vi "Calulate Rotation and Inclination.vi"(0 "Ch 0":dbl, 7 "Ch 1":dbl, 9 "Ch 2":dbl) -> (4 "Magnitude XYZ(g)":dbl, 8 "Inclination":dbl, 10 "Rotation":dbl)   [LabVIEW 2011]
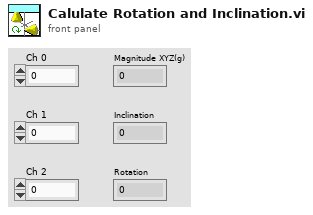
[diagram p1: front panel]
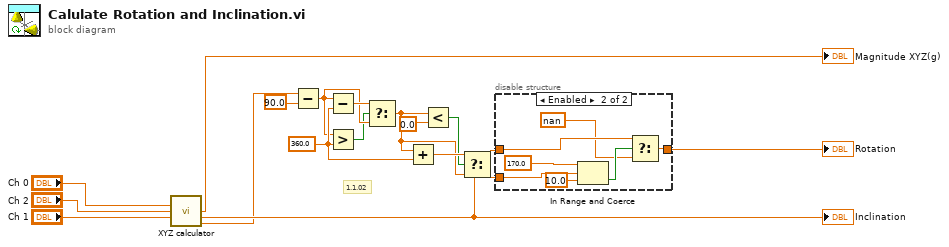
[diagram p0: block diagram]
diagram:
  w14 = 360.0 ("y")
  # "1.1.02"
  n1 = call "XYZ calculator.vi"("X(g)"="Ch 0", "Y(g)"="Ch 2", "Z(g)"="Ch 1") -> ("Magnitude XYZ(g)"=→"Magnitude XYZ(g)":dbl, "Angle z-xyz"=w7:dbl, "Angle x - xy w sign"=w4:dbl)  [unwired: 8 in, 2 out]
  "Inclination" <- w7
  n2 = Subtract(x=w4, y=90.0 ("x")) -> (x-y=w12:dbl)
  n3 = Subtract(x=w12, y=w14) -> (x-y=w13:dbl)
  n4 = Greater?(x=w12, y=w14) -> (0:w10:bool)
  n5 = Select(t=w13, s=w10, f=w12) -> (s? t:f=w15:dbl)
  n6 = Add(x=w15, y=w14) -> (x+y=w16:dbl)
  n7 = Less?(x=w15, y=0.0) -> (x < y?=w11:bool)
  n8 = Select(t=w16, s=w11, f=w15) -> (s? t:f=w17:dbl)
  n9 = disable-structure shown="Enabled" {
    disable-tunnel: w17 -> [w18 w20]
    disable-tunnel: [w18 w22] -> w5
    disable-tunnel: w7 -> [_ w25]
    frame Disabled {
    }
    frame Enabled {
      n10 = In Range and Coerce(upper limit=170.0, x=w25, lower limit=10.0) -> (In Range?=w21:bool)  [unwired: 1 out]
      n11 = Select(t=w20, s=w21, f=nan) -> (s? t:f=w22:dbl)
    }
  }
  "Rotation" <- w5
